vi "MapTesting.vi"() -> ()   [LabVIEW 2013]
uses:
  <vilib>/robotics/Navigation/shared/WorldMap/OccupancyGridWorldMap/NI_Robotics_OccupancyGridWorldMap.lvclass
panel:
  in  "Random?":bool
  in  "y":i32 min=0
  in  "x":i32
  in  "% Random Obstacles":dbl=40.0 min=0.0 max=100.0 step=1.0 format="%#_3g"
  in  "dimension size":i32=250
  in  "stop":bool
  out "path on obstacles":dbl[][](graph)
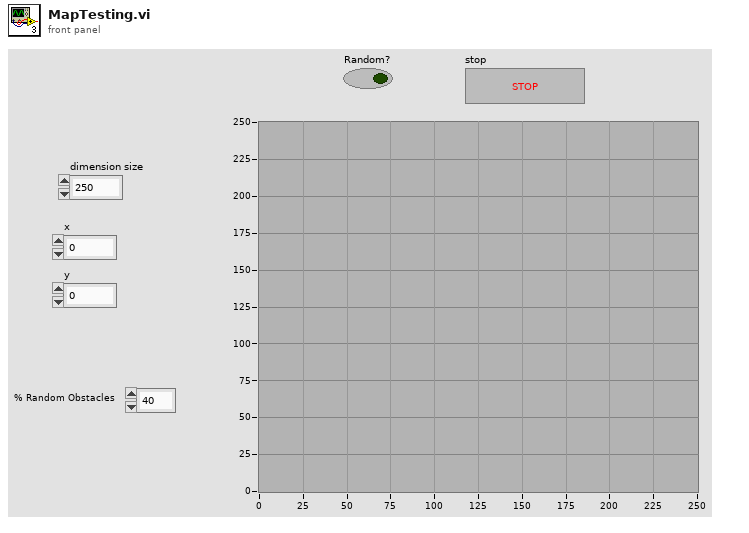
[diagram p1: front panel]
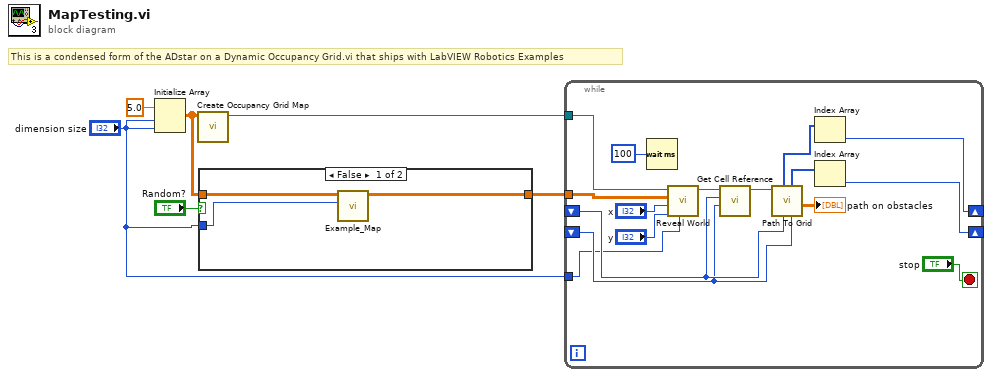
[diagram p0: block diagram]
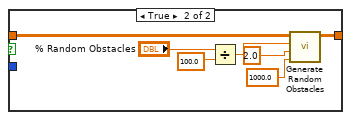
[diagram p2: hidden frame]
diagram:
  # "This is a condensed form of the ADstar on a Dynamic Occupancy Grid.vi that ships with LabVIEW Robotics Examples"
  n1 = Initialize Array(5.0 ("element"), "dimension size", "dimension size") -> (w6:dbl[][])
  n2 = call <vilib>:"Create Occupancy Grid Map.vi"("occupancy grid"=w6) -> ("map reference out"=w4:refnum<data-value>)  [unwired: 9 in, 1 out]
  n3 = case shown="False" "Random?" {
    tunnel: w6 -> [w9 w11]
    tunnel: [w8 w10] -> w3
    tunnel: "dimension size" -> [w7 _]
    frame False {
      n4 = call "Example_Map.vi"("dimension size"=w7, "Array in"=w9) -> ("Array out"=w8:dbl[][])  [unwired: 9 in]
    }
    frame True {
      n5 = Divide(x="% Random Obstacles", y=100.0) -> (x/y=w14:dbl)
      n6 = call "Generate Random Obstacles.vi"("obstacle cost"=1000.0, "free cost"=2.0, "chance"=w14, "cost in"=w11) -> ("cost out"=w10:dbl[][])  [unwired: 7 in]
    }
  }
  n7 = while {
    shift-right: [w26] -> _
    shift-left: _ -> [w21]
    shift-right: [w24] -> _
    shift-left: _ -> [w20]
    tunnel: w4 -> [w19]
    tunnel: w3 -> [w18]
    tunnel: "dimension size" -> [w17]
    stop <- "stop" stop-if-true
    n8 = Wait (ms)(milliseconds to wait=u32 100) -> ()  [unwired: 1 out]
    n9 = call "Reveal World.vi"("radius"=w17, "y"="y", "x"="x", "cost in"=w18, "map reference in"=w19) -> ("map reference in 2"=w30:refnum<data-value>)  [unwired: 5 in, 1 out]
    n10 = call <vilib>:"Get Cell Reference.vi"("y"=w20, "x"=w21, "map reference in"=w30) -> ("map reference out"=w29:refnum<data-value>)  [unwired: 5 in, 3 out]
    n11 = call "Path To Grid.vi"("current y"=w20, "current x"=w21, "map reference in"=w29) -> ("path on obstacles"=→"path on obstacles":dbl[][], "y coordinates"=w25:i32[], "x coordinates"=w27:i32[])  [unwired: 4 in, 2 out]
    n12 = Index Array(array=w27) -> (element=w26:i32)  [unwired: 1 in]
    n13 = Index Array(array=w25) -> (element=w24:i32)  [unwired: 1 in]
  }
